vi "배열만들기.vi"() -> ()   [LabVIEW 2014]
panel:
  out "x+y":dbl[][](array[numeric])=[[1.0, 1.0, 1.0], [1.0, 1.0, 1.0], [1.0, 1.0, 23.0]]
  in  "배열":dbl[][](array[numeric])=[[0.0, 0.0, 0.0], [0.0, 0.0, 0.0], [0.0, 0.0, 22.0]]
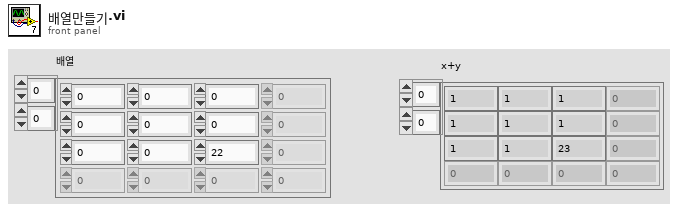
[diagram p1: front panel]
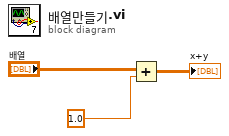
[diagram p0: block diagram]
diagram:
  n1 = Add(x="배열", y=1.0) -> (x+y=→"x+y":dbl[][])
